vi "Select Datatype.vi"(10 "data":string[](array[string]), 11 "Devicetype":string) -> (3 "Datatype":string[](array[string]))   [LabVIEW 2020]
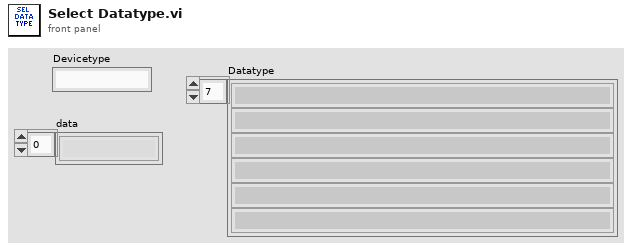
[diagram p1: front panel]
types:
  T1 = typedef "mysql_authentication.ctl" = cluster{"User":string, "Password":string, "Database":string}
  T2 = cluster{"Port":u16, "IP Address":string, "Authentication":T1}
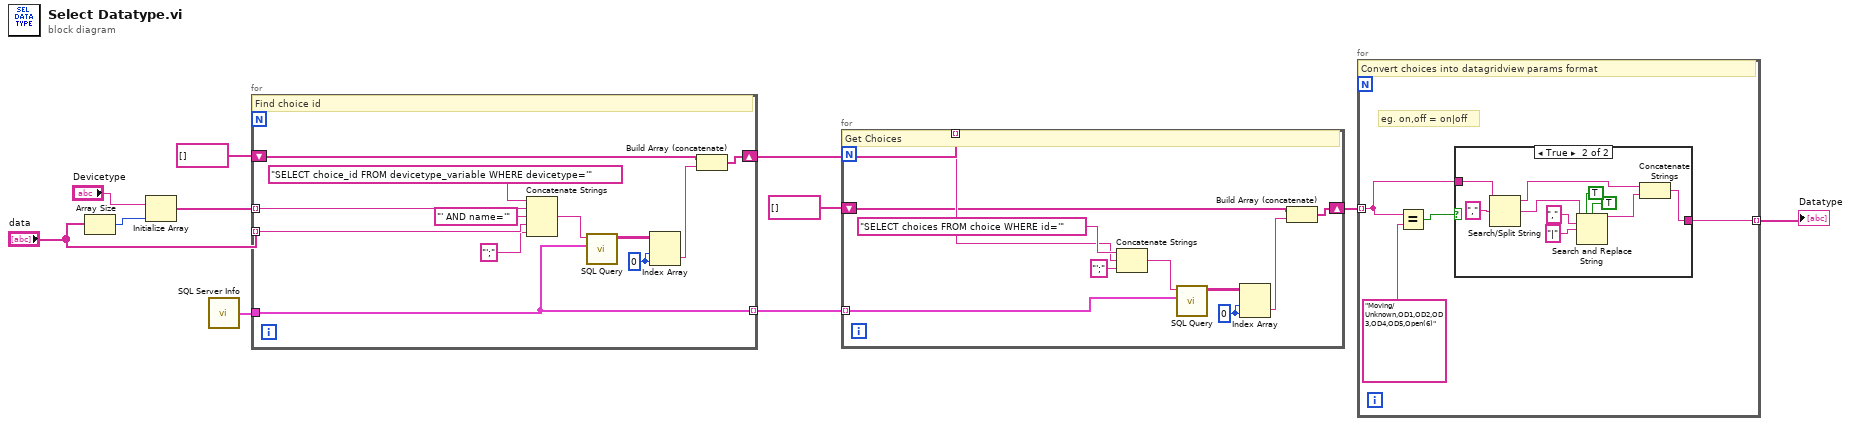
[diagram p0: block diagram]
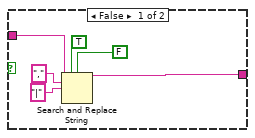
[diagram p2: hidden frame]
diagram:
  n1 = Array Size(array="data") -> (size(s)=w3:i32)
  n2 = Initialize Array("Devicetype", w3) -> (w1:string[])
  n3 = call "SQL Server Info.vi"() -> ("SQL Server Info"=w5:T2)
  n4 = for {
    shift-right: [w17] -> w8
    shift-left: string[] [] -> [w19]
    tunnel: w1 -> [w16] mode=indexing
    tunnel: w5 -> [w12]
    tunnel: "data" -> [w14] mode=indexing
    tunnel: [w12] -> w9 mode=indexing
    w20 = 0 ("disabled index (col)")
    # "Find choice id"
    n5 = Concatenate Strings("SELECT choice_id FROM devicetype_variable WHERE devicetype='", w16, "' AND name='" ("string"), w14, "';" ("string")) -> (w22:string)
    n6 = call "SQL Query.vi"("SQL Server Info"=w12, "Query"=w22) -> ("data"=w21:string[][])  [unwired: 8 in, 1 out]
    n7 = Index Array(array=w21, index (row)=w20, index (col)=w20) -> (element=w18:string)
    n8 = Build Array (concatenate)(w19, w18) -> (w17:string[])
  }
  n9 = for {
    tunnel: w8 -> [w28] mode=indexing
    shift-right: [w25] -> w10
    shift-left: string[] [] -> [w27]
    tunnel: w9 -> [w24] mode=indexing
    w29 = 0 ("disabled index (col)")
    # "Get Choices"
    n10 = Concatenate Strings("SELECT choices FROM choice WHERE id='", w28, "';" ("string")) -> (w31:string)
    n11 = call "SQL Query.vi"("SQL Server Info"=w24, "Query"=w31) -> ("data"=w30:string[][])  [unwired: 8 in, 1 out]
    n12 = Index Array(array=w30, index (row)=w29, index (col)=w29) -> (element=w26:string)
    n13 = Build Array (concatenate)(w27, w26) -> (w25:string[])
  }
  n14 = for {
    tunnel: w10 -> [w35] mode=indexing
    tunnel: [w34] -> w11 mode=indexing
    # "eg. on,off = on|off"
    # "Convert choices into datagridview params format"
    n15 = Equal?(x=w35, y="Moving/Unknown,OD1,OD2,OD3,OD4,OD5,Open(6)") -> (x = y?=w36:bool)
    n16 = case shown="True" w36 {
      tunnel: [w39 w45] -> w34
      tunnel: w35 -> [w38 w49]
      frame False {
        n17 = Search and Replace String(replace all?=TRUE ("replace all? (F)"), case sensitive?=FALSE ("ignore case? (F)"), input string=w38, search string=",", replace string="|" ("replace string (\"\")")) -> (result string=w39:string)  [unwired: 3 in, 3 out]
      }
      frame True {
        n18 = Search/Split String(string=w49, search string/char (-)=",") -> (substring before match=w44:string, match + rest of string=w47:string)  [unwired: 1 in, 1 out]
        n19 = Search and Replace String(replace all?=TRUE ("replace all? (F)"), case sensitive?=TRUE ("ignore case? (F)"), input string=w47, search string=",", replace string="|" ("replace string (\"\")")) -> (result string=w46:string)  [unwired: 3 in, 3 out]
        n20 = Concatenate Strings(w44, w46) -> (w45:string)
      }
    }
  }
  "Datatype" <- w11
